vi "issue_parser_tester.vi"() -> ()   [LabVIEW 2024]
uses:
  WebScraper/comic_class/comic_class.lvclass
  WebScraper/comic_class/comic_class.lvclass/comic_class.ctl
panel:
  out "last modified":timestamp
  in  "url":string
  out "error out":errorcluster
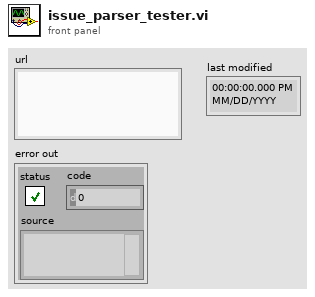
[diagram p1: front panel]
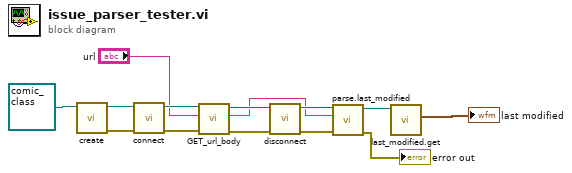
[diagram p0: block diagram]
diagram:
  n1 = call "create.vi"("comic_class in"=refnum<class "comic_class.lvclass"> refnum ("comic_class.lvclass")) -> ("error out"=w11:errorcluster, "comic_class out"=w14:refnum<class "comic_class.lvclass">)  [unwired: 9 in]
  n2 = call-dynamic "connect.vi"("error in (no error)"=w11, "comic_class in"=w14) -> ("error out"=w10:errorcluster, "comic_class out"=w13:refnum<class "comic_class.lvclass">)  [unwired: 8 in]
  n3 = call-dynamic "GET_url_body.vi"("error in (no error)"=w10, "url"="url", "comic_class in"=w13) -> ("error out"=w9:errorcluster, "body"=w4:string, "comic_class out"=w12:refnum<class "comic_class.lvclass">)  [unwired: 6 in]
  n4 = call-dynamic "disconnect.vi"("error in (no error)"=w9, "comic_class in"=w12) -> ("error out"=w6:errorcluster, "comic_class out"=w7:refnum<class "comic_class.lvclass">)  [unwired: 8 in]
  n5 = call-dynamic "parse.last_modified.vi"("error in (no error)"=w6, "body"=w4, "comic_class in"=w7) -> ("error out"=→"error out":errorcluster, "comic_class out"=w2:refnum<class "comic_class.lvclass">)  [unwired: 7 in]
  n6 = call "last_modified.get.vi"("comic_class in"=w2) -> ("last modified"=→"last modified":timestamp)  [unwired: 9 in, 1 out]
